vi "Get Finger Positions.vi"(8 "error in (no error)":errorcluster, 11 "MF3 in":refnum<class "MF3.lvclass">) -> (0 "error out":errorcluster, 2 "Finger Positions":T1, 3 "MF3 out":refnum<class "MF3.lvclass">)   [LabVIEW 2011, in "MF3.lvclass"]
uses:
  MF3.lvclass
  MF3.lvclass/MF3.ctl
  Finger/Finger.lvclass
  <vilib>/robotics/Kinematics/NI_Kinematics.lvlib
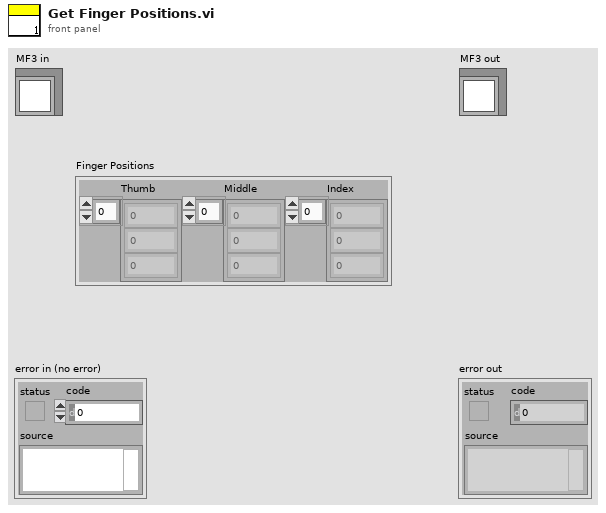
[diagram p1: front panel]
types:
  T1 = cluster{"Thumb":dbl[], "Middle":dbl[], "Index":dbl[]}
  T2 = typedef "NI_Matrix.lvlib/RealMatrix.ctl" = dbl[][]
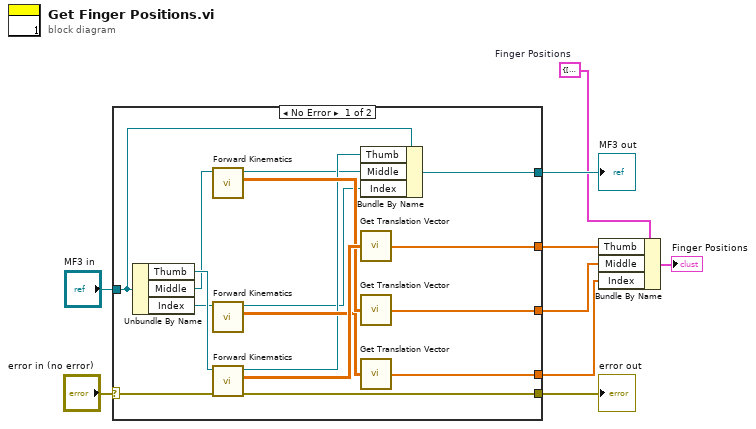
[diagram p0: block diagram]
diagram:
  w5 = T1 {"Thumb"=[], "Middle"=[], "Index"=[]}  # Finger Positions
  n1 = case shown="No Error" "error in (no error)" {
    selector: "error in (no error)" -> [w24 w27]
    tunnel: [w23 w27] -> w8
    tunnel: [w10 w26] -> w6
    tunnel: "MF3 in" -> [w14 w26]
    tunnel: [w21 _] -> w3
    tunnel: [w17 _] -> w2
    tunnel: [w15 _] -> w1
    frame No Error {
      n2 = Unbundle By Name(w14) -> ("Thumb"=w25:refnum<class "Finger.lvclass">, "Middle"=w20:refnum<class "Finger.lvclass">, "Index"=w19:refnum<class "Finger.lvclass">)
      n3 = call "Forward Kinematics.vi"("Finger in"=w20) -> ("T"=w18:T2, "Finger out"=w12:refnum<class "Finger.lvclass">)  [unwired: 8 in, 1 out]
      n4 = call "Forward Kinematics.vi"("Finger in"=w19) -> ("T"=w16:T2, "Finger out"=w11:refnum<class "Finger.lvclass">)  [unwired: 8 in, 1 out]
      n5 = call "Forward Kinematics.vi"("error in (no error)"=w24, "Finger in"=w25) -> ("error out"=w23:errorcluster, "T"=w22:T2, "Finger out"=w13:refnum<class "Finger.lvclass">)  [unwired: 7 in]
      n6 = Bundle By Name(cluster=w14, "Thumb"=w13, "Middle"=w12, "Index"=w11) -> (w10:refnum<class "MF3.lvclass">)
      n7 = call <vilib>:"Get Translation Vector.vi"("transform"=w22) -> ("translation vector"=w21:dbl[])
      n8 = call <vilib>:"Get Translation Vector.vi"("transform"=w18) -> ("translation vector"=w17:dbl[])
      n9 = call <vilib>:"Get Translation Vector.vi"("transform"=w16) -> ("translation vector"=w15:dbl[])
    }
    frame Error {
    }
  }
  "error out" <- w8
  "MF3 out" <- w6
  n10 = Bundle By Name(cluster=w5, "Thumb"=w3, "Middle"=w2, "Index"=w1) -> (→"Finger Positions":T1)
